vi "Read ListItems.vi"(8 "error in (no error)":errorcluster, 11 "ScrollingList in":refnum<class "ScrollingList.lvclass">) -> (0 "error out":errorcluster, 2 "List Items":string[](array[string]), 3 "ScrollingList out":refnum<class "ScrollingList.lvclass">)   [LabVIEW 2020, in "ScrollingList.lvclass"]
uses:
  ScrollingList.lvclass
  ScrollingList.lvclass/ScrollingList.ctl
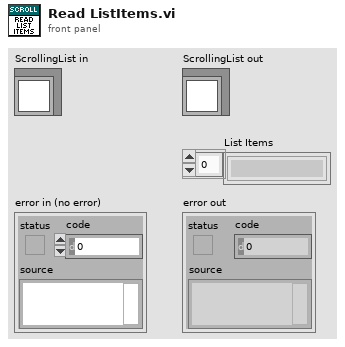
[diagram p1: front panel]
types:
  T1 = typedef "ScrollingList.lvclass/State Data.ctl" = cluster{"Timeout":i32, "Time":timestamp, "Y":i32, "Origin:Top":i16, "Rate":dbl, "ListItems":string[], "Item Height":i32, "Max Height":i32}
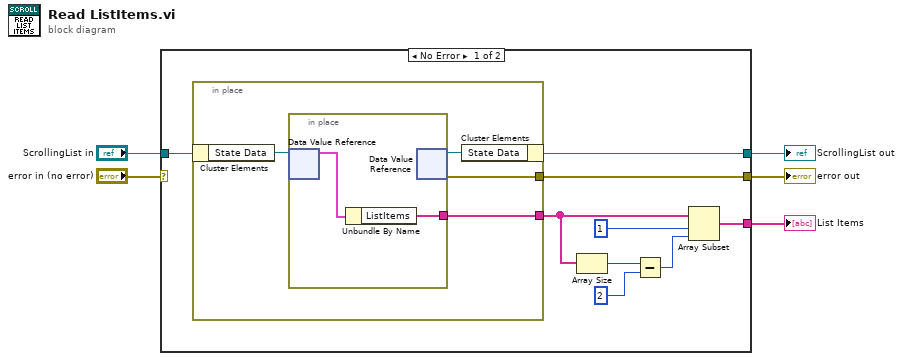
[diagram p0: block diagram]
diagram:
  n1 = case shown="No Error" "error in (no error)" {
    selector: "error in (no error)" -> [_ w22]
    tunnel: [w13 w22] -> w4
    tunnel: [w12 w21] -> w2
    tunnel: "ScrollingList in" -> [w14 w21]
    tunnel: [w9 _] -> w1
    frame No Error {
      n2 = in-place {
        in-place-border: [w16] -> w13
        in-place-border: [w15] -> w10
        n3 = in-place-cluster #1(w14) -> ("State Data"=w18:refnum<data-value>)
        n4 = in-place {
          in-place-border: [w19] -> w15
          n5 = in-place-dvr #2(w18) -> (w20:T1)  [unwired: 1 out]
          n6 = Unbundle By Name(w20) -> ("ListItems"=w19:string[])
          n7 = in-place-dvr #2() -> (w17:refnum<data-value>, w16:errorcluster)  [unwired: 1 in]
        }
        n8 = in-place-cluster #1("State Data"=w17) -> (w12:refnum<class "ScrollingList.lvclass">)
      }
      n9 = Array Size(array=w10) -> (size(s)=w8:i32)
      n10 = Subtract(x=w8, y=2) -> (x-y=w7:i32)
      n11 = Array Subset(array=w10, index=1, length=w7) -> (w9:string[])
    }
    frame Error {
    }
  }
  "error out" <- w4
  "ScrollingList out" <- w2
  "List Items" <- w1
